vi "PIDTEMPtest.vi"() -> ()   [LabVIEW 2015]
uses:
  <vilib>/DAQmx/read.llb/DAQmx Read (Analog 1D Wfm NChan 1Samp).vi
  <vilib>/Analysis/baseanly.llb/Mean (DBL).vi
  <vilib>/DAQmx/write.llb/DAQmx Write (Digital 1D Bool NChan 1Samp 1Line).vi
  <vilib>/DAQmx/miscellaneous.llb/DAQmx Fill In Error Info.vi
  <vilib>/addons/control/pid/pid.llb/PID Advanced (DBL).vi
  <vilib>/Utility/file.llb/Write Delimited Spreadsheet (DBL).vi
  <vilib>/addons/control/pid/NI_PID_pid.lvlib
  <vilib>/Analysis/NI_AALBase.lvlib
panel:
  out "Temp":dbl
  out "Numeric 3":i32
  out "Numeric":i32
  in  "Duty Cycle %":dbl
  in  "reinitialize? (F)":bool
  in  "relative max cycle time (s)":dbl=0.01
  out "Voltage Reading(Temp)":dbl format="%#_13g"
  out "Temperature (Celcius)":dbl format="%#.1g"
  out "Temp(C)":dbl(slide) scale=-10.0..100.0
  out "Temp Chart":waveform(dbl)(graph)
  out "Temp Chart 2":waveform(dbl)(graph)
  in  "Temp Setting":dbl
  in  "PID gains Temp":T1={"proportional gain (Kc)"=1.0, "integral time (Ti, min)"=0.01, "derivative time (Td, min)"=0.0} {"derivative time (Td, min)" format="%.3f"; "integral time (Ti, min)" format="%.3f"; "proportional gain (Kc)" format="%.3f"}
  in  "Stop Maintaining Temp":bool
  out "Control Value (Temp Sensor)":dbl(knob) scale=0.0..100.0
  out "Heater On/off":bool
  out "Cycle time  from Control Value":dbl
  in  "Steps in a cycle":i32=256
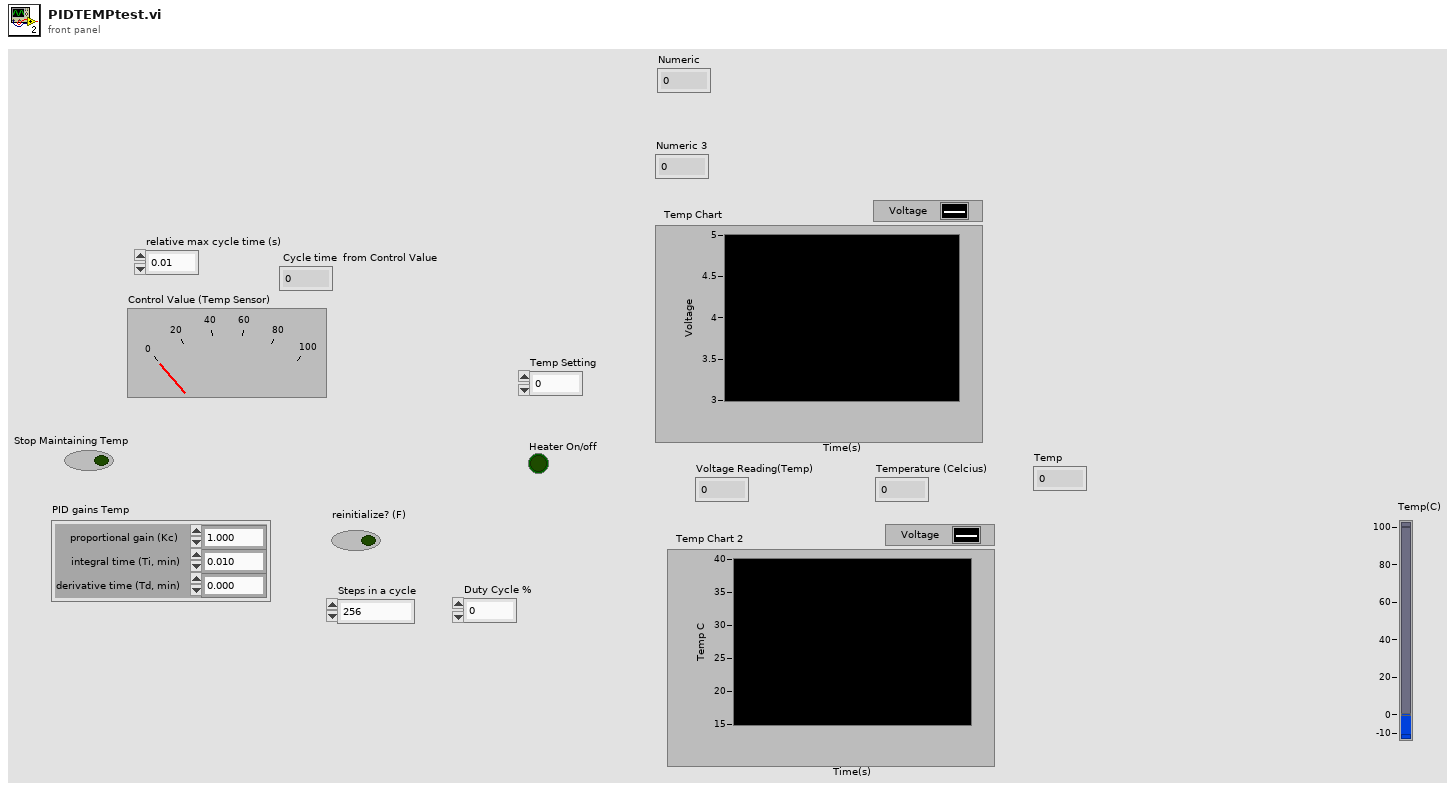
[diagram p1: front panel]
types:
  T1 = cluster{"proportional gain (Kc)":dbl, "integral time (Ti, min)":dbl, "derivative time (Td, min)":dbl}
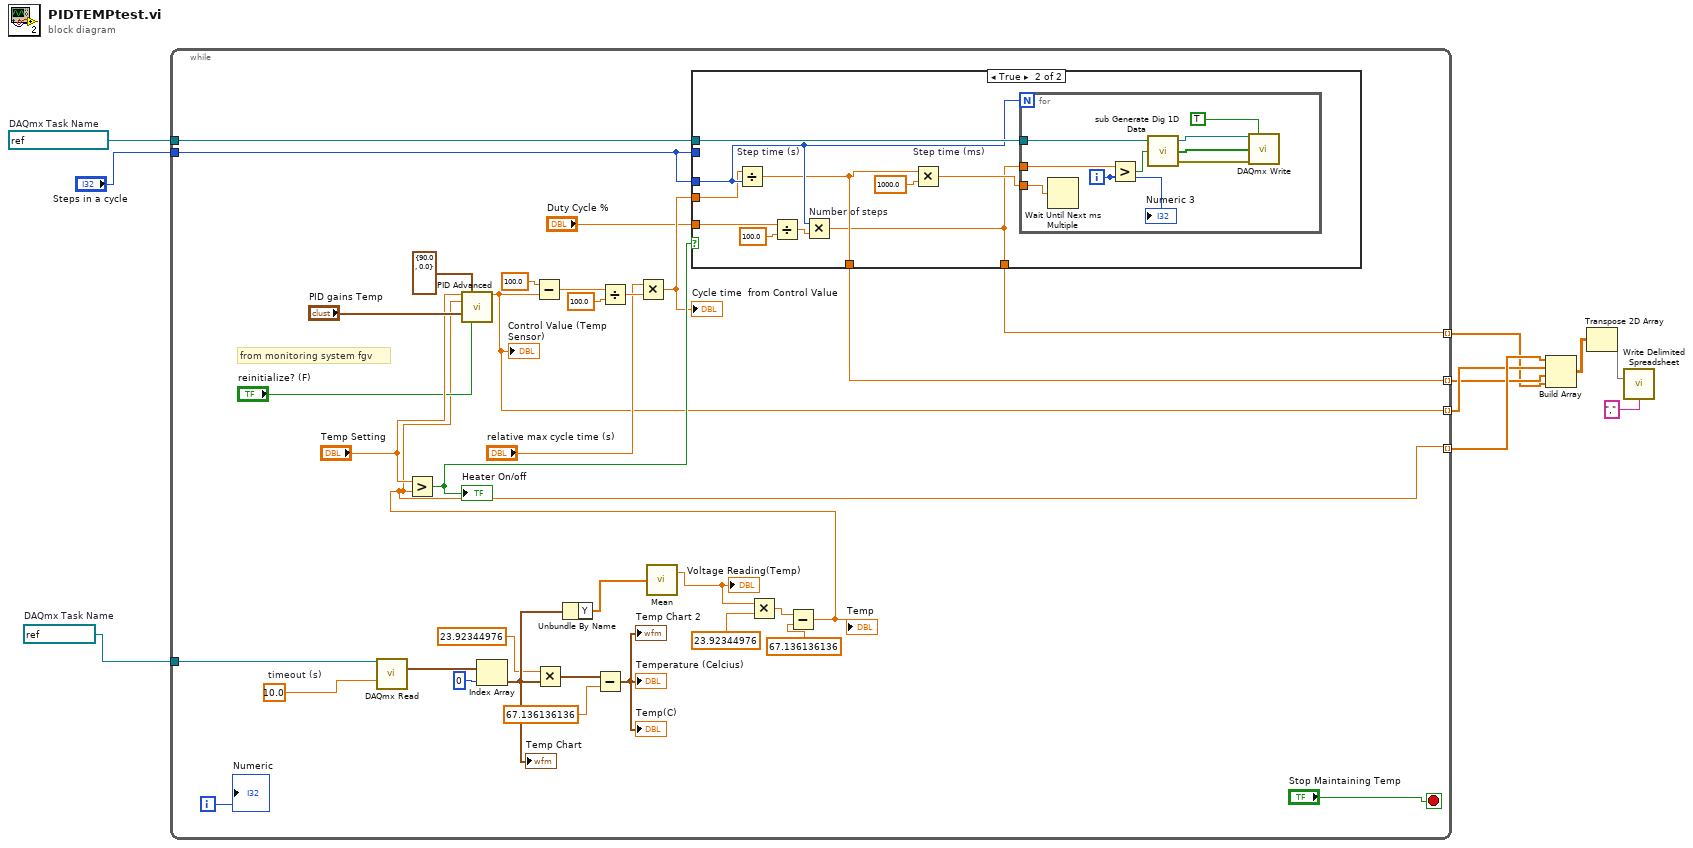
[diagram p0: block diagram]
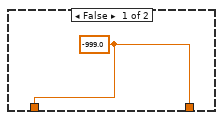
[diagram p2: hidden frame]
diagram:
  w1 = refnum<k21> "A0New1"  # DAQmx Task Name
  w10 = refnum<k21> "P0L0DigitalOut"  # DAQmx Task Name
  n1 = while {
    tunnel: w10 -> [w44]
    tunnel: "Steps in a cycle" -> [w42]
    tunnel: [w29] -> w5 mode=indexing
    tunnel: [w28] -> w6 mode=indexing
    tunnel: [w27] -> w7 mode=indexing
    tunnel: [w11] -> w8 mode=indexing
    tunnel: w1 -> [w12]
    i -> [w26]
    stop <- "Stop Maintaining Temp" stop-if-true
    w13 = 10.0  # timeout (s)
    # "from monitoring system fgv"
    n2 = call-poly <vilib>:"DAQmx Read.vi"("task/channels in"=w12, "timeout"=w13) -> ("data"=w18:waveform(dbl)[])  [unwired: 11 in, 2 out]
    n3 = Index Array(array=w18, index=0) -> (element=w20:waveform(dbl))
    "Temp Chart" <- w20
    n4 = Multiply(x=23.92344976, y=w20) -> (x*y=w15:waveform(dbl))
    n5 = Unbundle By Name(w20) -> ("Y"=w21:dbl[])
    n6 = Subtract(x=w15, y=67.136136136) -> (x-y=→"Temperature (Celcius)" →"Temp(C)" →"Temp Chart 2":waveform(dbl))
    n7 = call-poly <vilib>:"Mean.vi"("X"=w21) -> ("mean"=w22:dbl)  [unwired: 1 out]
    "Voltage Reading(Temp)" <- w22
    n8 = Multiply(x=w22, y=23.92344976) -> (x*y=w23:dbl)
    n9 = Subtract(x=w23, y=67.136136136) -> (x-y=w11:dbl)
    "Temp" <- w11
    n10 = Greater?(x="Temp Setting", y=w11) -> (0:w41:bool)
    "Heater On/off" <- w41
    n11 = call-poly <vilib>:"PID Advanced.vi"("setpoint"="Temp Setting", "output range"=cluster{"output high":dbl, "output low":dbl} {"output high"=90.0, "output low"=0.0}, "process variable"=w11, "PID gains"="PID gains Temp", "reinitialize? (F)"="reinitialize? (F)") -> ("output"=w27:dbl)  [unwired: 9 in, 1 out]
    "Control Value (Temp Sensor)" <- w27
    n12 = Subtract(x=100.0, y=w27) -> (x-y=w34:dbl)
    n13 = Divide(x=w34, y=100.0) -> (x/y=w35:dbl)
    n14 = Multiply(x="relative max cycle time (s)", y=w35) -> (x*y=w36:dbl)
    "Cycle time  from Control Value" <- w36
    n15 = case shown="True" w41 {
      tunnel: w44 -> [_ w55]
      tunnel: w36 -> [_ w50]
      tunnel: w42 -> [_ w51]
      tunnel: "Duty Cycle %" -> [_ w52]
      tunnel: w42 -> [_ _]
      tunnel: [w45 w47] -> w28
      tunnel: [w45 w46] -> w29
      frame False {
        w45 = -999.0
      }
      frame True {
        n16 = Divide "Step time (s)"(x=w50, y=w51) -> (x/y=w47:dbl)
        n17 = Divide(x=w52, y=100.0) -> (x/y=w53:dbl)
        n18 = Multiply "Number of steps"(x=w51, y=w53) -> (x*y=w46:dbl)
        n19 = Multiply "Step time (ms)"(x=w47, y=1000.0) -> (x*y=w48:dbl)
        n20 = for {
          N: w51 -> [_]
          tunnel: w55 -> [w61]
          tunnel: w46 -> [w60]
          tunnel: w48 -> [w56]
          i -> [w59]
          n21 = Wait Until Next ms Multiple(millisecond multiple=w56) -> ()  [unwired: 1 out]
          n22 = Greater?(x=w60, y=w59) -> (0:w57:bool)
          n23 = call <vilib>:"sub Generate Dig 1D Data.vi"("initial value"=w57, "task in"=w61) -> ("error out"=w63:errorcluster, "Data"=w58:bool[], "task out"=w62:refnum<k21>)  [unwired: 1 in]
          n24 = call-poly <vilib>:"DAQmx Write.vi"("task/channels in"=w62, "auto start"=TRUE, "data"=w58, "error in"=w63) -> ()  [unwired: 9 in, 3 out]
          "Numeric 3" <- w59
        }
      }
    }
    "Numeric" <- w26
  }
  n25 = Build Array(w8, w7, w6, w5) -> (w4:dbl[][])
  n26 = Transpose 2D Array(2D array=w4) -> (transposed array=w2:dbl[][])
  n27 = call-poly <vilib>:"Write Delimited Spreadsheet.vi"("2D data"=w2, "delimiter (\\t)"="," ("delimiter (\\t)")) -> ()  [unwired: 12 in, 2 out]
